vi "Read Measurement Units.vi"(7 "Unit ID (A)":string="A", 8 "error in":errorcluster, 10 "Software Rev":u8, 11 "VISA Session In":refnum<visa-resource-name>="Alicat") -> (0 "error out":errorcluster, 1 "Lock Gas Select":bool, 2 "Measurement Units":T2, 3 "VISA Session Out":refnum<visa-resource-name>)   [LabVIEW 2016]
doc: "Reads the measurement units for the available variables. Measurement units are returned as strings."
uses:
  Omega FMA-1600A Series Gas Flow Meter/Type Definitions/FMA1600A Units String.ctl
  Omega FMA-1600A Series Gas Flow Meter/Type Definitions/FMA1600A Units.ctl
panel:
  in  "Gauge (T) or \nDifferential (F)":bool
  out "Measurement Units Intermediate\n(newer revisions)":T1={"Abs. Pressure Units"=1, "Gauge/Diff. Press. Units"=1, "Barometric Press. Units"=1, "Temperature Units"=1, "Volumetric Units"=1, "Mass Units"=1, "Setpoint Units"=1, "Valve Drive Units"=1, "Total Mass Units"=1, "Total Volume Units"=1, "Time Units"=1} {"Setpoint Units" items=["Default"=0, "Unknown"=1, "SuL/m"=2, "SmL/s"=3, "SmL/m"=4, "SmL/h"=5, "SL/s"=6, "SLPM"=7, "SL/h"=8, "SCCS"=11, "SCCM"=12, "Scm3/h"=13, "Sm3/m"=14, "Sm3/h"=15, "Sm3/d"=16, "Sin3/m"=17, "SCFM"=18, "SCFH"=19, "kSCFM"=20, "NuL/m"=32, "NmL/s"=33, "NmL/m"=34, "NmL/h"=35, "NL/s"=36, "NLPM"=37, "NL/h"=38, "NCCS"=41, "NCCM"=42, "Ncm3/h"=43, "Nm3/m"=44, "Nm3/h"=45, "Nm3/d"=46, "count"=62, "%"=63, "mg/s"=64, "mg/m"=65, "g/s"=66, "g/m"=67, "g/h"=68, "kg/m"=69, "kg/h"=70, "oz/s"=71, "oz/m"=72, "lb/m"=73, "lb/h"=74]; "Barometric Press. Units" items=["Default"=0, "Unknown"=1, "Pa"=2, "hPa"=3, "kPa"=4, "MPa"=5, "mbar"=6, "bar"=7, "g/cm2"=8, "kg/cm"=9, "PSI"=10, "PSF"=11, "mTorr"=12, "torr"=13, "mmHg"=14, "inHg"=15, "mmH2O"=16, "mmH2O"=17, "cmH2O"=18, "cmH2O"=19, "inH2O"=20, "inH2O"=21, "atm"=22, "m asl"=23, "ft asl"=24, "V"=61, "count"=62, "%"=63]; "Gauge/Diff. Press. Units" items=["Default"=0, "Unknown"=1, "Pa"=2, "hPa"=3, "kPa"=4, "MPa"=5, "mbar"=6, "bar"=7, "g/cm2"=8, "kg/cm"=9, "PSI"=10, "PSF"=11, "mTorr"=12, "torr"=13, "mmHg"=14, "inHg"=15, "mmH2O"=16, "mmH2O"=17, "cmH2O"=18, "cmH2O"=19, "inH2O"=20, "inH2O"=21, "atm"=22, "m asl"=23, "ft asl"=24, "V"=61, "count"=62, "%"=63]; "Time Units" items=["Default", "Unknown", "h:m:s", "ms", "s", "m", "hour", "day"]; "Total Volume Units" items=["Default"=0, "Unknown"=1, "uL"=2, "mL"=3, "L"=4, "US GAL"=5, "cm3"=6, "m3"=7, "in3"=8, "ft3"=9, "uP"=61]; "Total Mass Units" items=["Default"=0, "Unknown"=1, "SuL"=2, "SmL"=3, "SL"=4, "Scm3"=6, "Sm3"=7, "Sin3"=8, "Sft3"=9, "kSft3"=10, "NuL"=32, "NmL"=33, "NL"=34, "Ncm3"=35, "Nm3"=36, "mg"=64, "g"=65, "kg"=66, "oz"=67, "lb"=68]; "Valve Drive Units" items=["Default"=0, "Unknown"=1, "count"=2, "%"=63]; "Mass Units" items=["Default"=0, "Unknown"=1, "SuL/m"=2, "SmL/s"=3, "SmL/m"=4, "SmL/h"=5, "SL/s"=6, "SLPM"=7, "SL/h"=8, "SCCS"=11, "SCCM"=12, "Scm3/h"=13, "Sm3/m"=14, "Sm3/h"=15, "Sm3/d"=16, "Sin3/m"=17, "SCFM"=18, "SCFH"=19, "kSCFM"=20, "NuL/m"=32, "NmL/s"=33, "NmL/m"=34, "NmL/h"=35, "NL/s"=36, "NLPM"=37, "NL/h"=38, "NCCS"=41, "NCCM"=42, "Ncm3/h"=43, "Nm3/m"=44, "Nm3/h"=45, "Nm3/d"=46, "count"=62, "%"=63, "mg/s"=64, "mg/m"=65, "g/s"=66, "g/m"=67, "g/h"=68, "kg/m"=69, "kg/h"=70, "oz/s"=71, "oz/m"=72, "lb/m"=73, "lb/h"=74]; "Volumetric Units" items=["Default"=0, "Unknown"=1, "uL/m"=2, "mL/s"=3, "mL/m"=4, "mL/h"=5, "L/s"=6, "LPM"=7, "L/h"=8, "US GPM"=9, "US GPH"=10, "CCS"=11, "CCM"=12, "cm3/h"=13, "m3/m"=14, "m3/h"=15, "m3/d"=16, "in3/m"=17, "CFM"=18, "CFH"=19, "count"=62, "%"=63]; "Temperature Units" items=["Default", "Unknown", "°C", "°F", "K", "°Ra"]; "Abs. Pressure Units" items=["Default"=0, "Unknown"=1, "Pa"=2, "hPa"=3, "kPa"=4, "MPa"=5, "mbar"=6, "bar"=7, "g/cm2"=8, "kg/cm"=9, "PSI"=10, "PSF"=11, "mTorr"=12, "torr"=13, "mmHg"=14, "inHg"=15, "mmH2O"=16, "mmH2O"=17, "cmH2O"=18, "cmH2O"=19, "inH2O"=20, "inH2O"=21, "atm"=22, "m asl"=23, "ft asl"=24, "V"=61, "count"=62, "%"=63]}
  out "Measurement Units Intermediate\n(older revisions)":T3={"Pressure Units"=0, "Mass Units"=0, "Temperature Units"=0, "Volume Units"=0, "Totalizer Units"=15, "Totalizer Avg Units"=15} {"Totalizer Units" items=["CC", "uL", "L", "CI", "CF", "CM", "GAL", "mL", "uP", "Lbs", "N/A", "N/A", "N/A", "SCC", "SuL", "SL", "SCI", "SCF", "NCM", "Grams", "Kg", "Lbs", "mg", "SCM", "SmL", "KSCF"]; "Totalizer Avg Units" items=["CCM", "uLPM", "LPM", "CIM", "CFM", "CM/M", "GAL/M", "mLPM", "uP/M", "Lbs/M", "N/A", "N/A", "N/A", "SCCM", "SuLPM", "SLPM", "SCIM", "SCFM", "NCM/M", "Grams/M", "Kg/M", "Lbs/M", "mg/M", "SCM/M", "SmLPM", "KSCFM"]; "Volume Units" items=["CCM"=0, "CCH"=64, "uLPM"=256, "LPS"=320, "LPM"=512, "CM/D"=576, "CIM"=768, "Percent"=832, "CFH"=1024, "Kg/M"=1088, "CM/H"=1280, "Kg/H"=1344, "CFM"=1536, "mLPS"=1600, "GPM"=1792, "CCS"=1856, "GPH"=2048, "mLPH"=2112, "Grams/S"=2304, "Lbs/H"=2368, "Grams/M"=2560, "Grams/H"=2816, "mg/M"=3072, "LPH"=3328, "oz/S"=3584, "mLPM"=3840]; "Temperature Units" items=["C"=0, "K"=16, "F"=32, "R"=48]; "Mass Units" items=["SCCM"=0, "SLPH"=128, "SuLPM"=4096, "SmLPM"=4224, "SLPM"=8192, "Grams/S"=8320, "SCIM"=12288, "SCM/H"=12416, "SCFH"=16384, "SCCH"=16512, "NCM/H"=20480, "NLPH"=20608, "SCFM"=24576, "NLPS"=24704, "Grams/M"=28672, "SCM/D"=28800, "Grams/H"=32768, "NmLPM"=32896, "Kg/M"=36864, "SCCS"=36992, "Kg/H"=40960, "NmLPH"=41088, "Lbs/M"=45056, "SLPS"=45184, "Lbs/H"=49152, "SmLPS"=49280, "mg/M"=53248, "mg/S"=53376, "NLPM"=57344, "NCCM"=61440]; "Pressure Units" items=["PSI", "PSI", "Torr", "Bar", "mBar", "Pascal", "KPa", "MPa", "inHg", "mmHg", "inH2O", "PSID", "mTorr", "cmH2O", "Kg/CM2", "mmH2O"]}
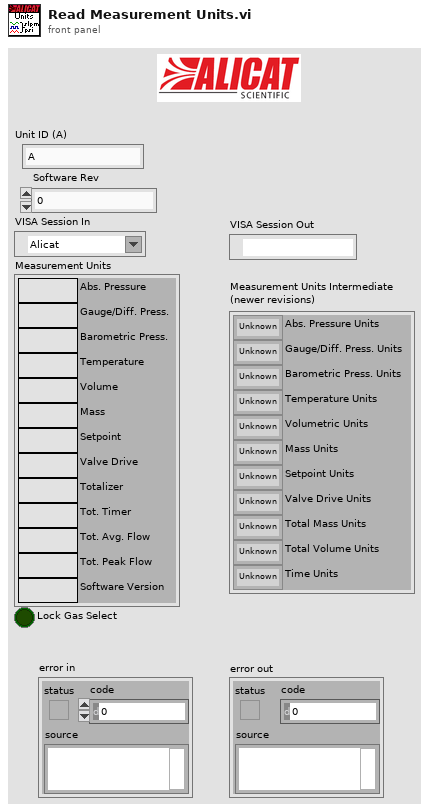
[diagram p1: front panel]
types:
  T1 = typedef "FMA1600A Units.ctl" = cluster{"Abs. Pressure Units":u16, "Gauge/Diff. Press. Units":u16, "Barometric Press. Units":u16, "Temperature Units":u16, "Volumetric Units":u16, "Mass Units":u16, "Setpoint Units":u16, "Valve Drive Units":u16, "Total Mass Units":u16, "Total Volume Units":u16, "Time Units":u16}
  T2 = typedef "FMA1600A Units String.ctl" = cluster{"Abs. Pressure":string, "Gauge/Diff. Press.":string, "Barometric Press.":string, "Temperature":string, "Volume":string, "Mass":string, "Setpoint":string, "Valve Drive":string, "Totalizer":string, "Tot. Timer":string, "Tot. Avg. Flow":string, "Tot. Peak Flow":string, "Software Version":string}
  T3 = cluster{"Pressure Units":i32, "Mass Units":i32, "Temperature Units":i32, "Volume Units":i32, "Totalizer Units":u16, "Totalizer Avg Units":u16}
  T4 = cluster{"Pressure":i32, "Mass":i32, "Temperature":i32, "Volume":i32, "Totalizer Units":u16, "Totalizer Avg Units":u16}
  T5 = typedef "LVStringsAndValuesArrayTypeDef_U16.ctl" = cluster{"String":string, "Value":u16}[]
  T6 = cluster{"Controller Select":u16, "SetPoint Source":enum8{"Serial", "Local", "Analog", "Unknown"}, "AutoTare":enum16{"Disabled", "Enabled"}}
  T7 = typedef "LVStringsAndValuesArrayTypeDef_I32.ctl" = cluster{"String":string, "Value":i32}[]
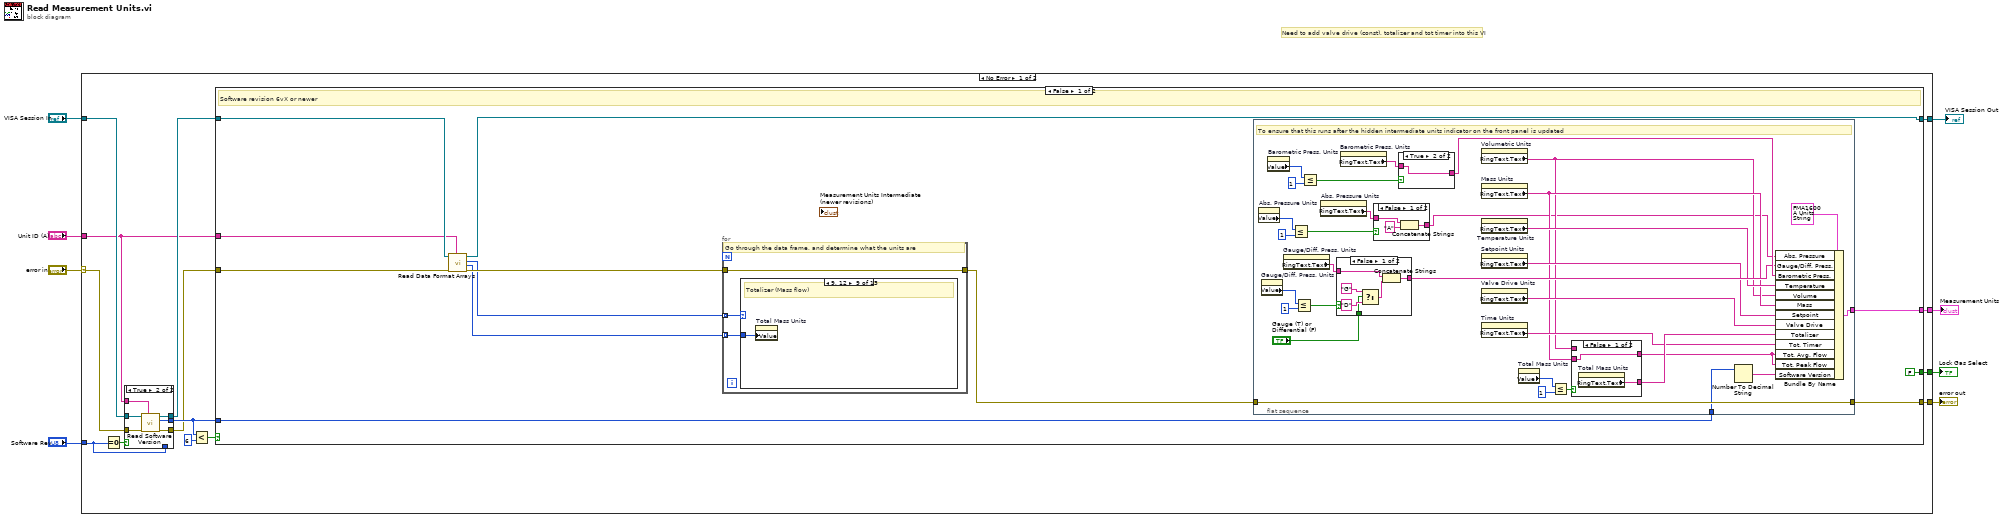
[diagram p0: block diagram]
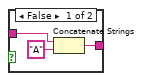
[diagram p4: hidden frame]
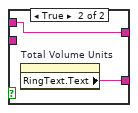
[diagram p6: hidden frame]
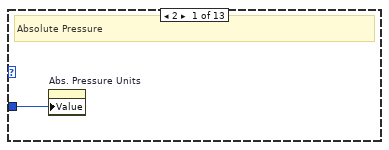
[diagram p7: hidden frame]
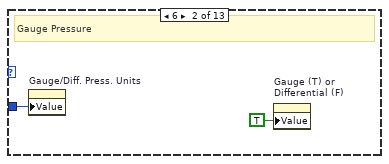
[diagram p8: hidden frame]
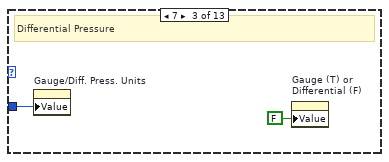
[diagram p9: hidden frame]
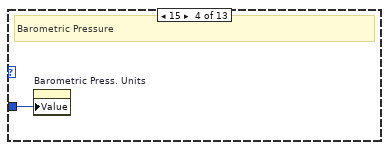
[diagram p10: hidden frame]
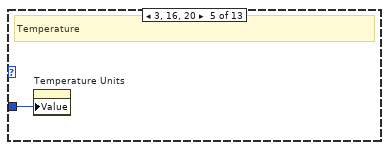
[diagram p11: hidden frame]
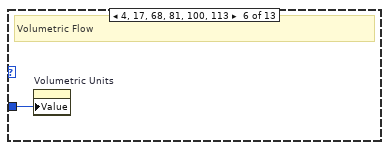
[diagram p12: hidden frame]
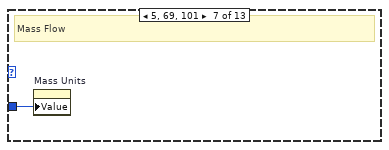
[diagram p13: hidden frame]
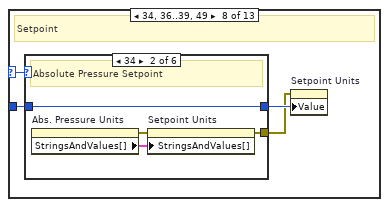
[diagram p14: hidden frame]
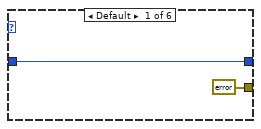
[diagram p15: hidden frame]
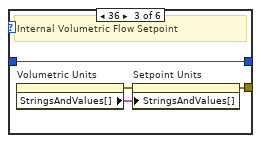
[diagram p16: hidden frame]
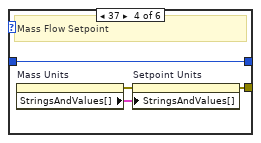
[diagram p17: hidden frame]
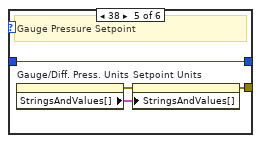
[diagram p18: hidden frame]
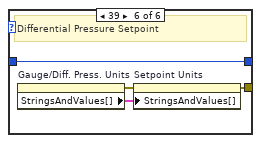
[diagram p19: hidden frame]
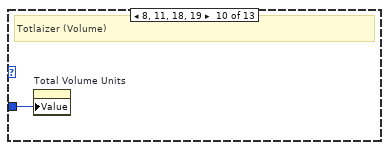
[diagram p20: hidden frame]
diagram:
  # "Need to add valve drive (const), totalizer and tot timer into this VI"
  n1 = case shown="No Error" "error in" {
    selector: "error in" -> [w11 w259]
    tunnel: [w22 TRUE ("Lock Gas Select")] -> w8
    tunnel: [w21 w259] -> w7
    tunnel: "Software Rev" -> [w15 _]
    tunnel: "Unit ID (A)" -> [w9 _]
    tunnel: "VISA Session In" -> [w10 w261]
    tunnel: [w19 w261] -> w3
    tunnel: [w18 T2 {"Abs. Pressure"="PSIA", "Gauge/Diff. Press."="Unknown", "Barometric Press."="Unknown", "Temperature"="°F", "Volume"="LPM", "Mass"="SLPM", "Setpoint"="Unknown", "Valve Drive"="Unknown", "Totalizer"="SL", "Tot. Timer"="Unknown", "Tot. Avg. Flow"="SLPM", "Tot. Peak Flow"="SLPM", "Software Version"=""} ("Measurement Units 2")] -> w2
    frame No Error {
      n2 = Equal To 0?(x=w15) -> (x = 0?=w16:bool)
      n3 = case shown="True" w16 {
        tunnel: w11 -> [w24 w31]
        tunnel: w10 -> [w23 w30]
        tunnel: w9 -> [_ w29]
        tunnel: [w24 w28] -> w12
        tunnel: [w23 w27] -> w13
        tunnel: [w25 w26] -> w14
        tunnel: w15 -> [w25 _]
        frame False {
        }
        frame True {
          n4 = call "Read Software Version.vi"("Unit ID (A)"=w29, "error in"=w31, "VISA Session In"=w30) -> ("error out"=w28:errorcluster, "Software Version"=w26:u8, "VISA Session Out"=w27:refnum<visa-resource-name>)  [unwired: 6 in]
        }
      }
      n5 = Less?(x=w14, y=u8 6) -> (x < y?=w20:bool)
      n6 = case shown="False" w20 {
        tunnel: [FALSE ("Lock Gas Select") w160] -> w22
        tunnel: w12 -> [w39 w152]
        tunnel: [w41 w147] -> w21
        tunnel: w14 -> [w32 w137]
        tunnel: w13 -> [w38 w153]
        tunnel: w9 -> [w37 w142]
        tunnel: [w36 w149] -> w19
        tunnel: [w40 w148] -> w18
        frame False {
          # "Software revision 6vX or newer"
          n7 = call "Read Data Format Arrays.vi"("Unit ID (A)"=w37, "error in (no error)"=w39, "VISA Session In"=w38) -> ("error out"=w35:errorcluster, "Units Array"=w33:u16[], "Data Type Array"=w34:u16[], "VISA Session Out"=w36:refnum<visa-resource-name>)  [unwired: 5 in]
          n8 = for {
            tunnel: w33 -> [w96] mode=indexing
            tunnel: w34 -> [w97] mode=indexing
            tunnel: [w95] -> w42
            tunnel: w35 -> [w95]
            # "Go through the data frame, and determine what the units are"
            n9 = case shown="9, 12" w97 {
              selector: w97 -> [_ _ _ _ _ _ _ w108 _ _ _ _ _]
              tunnel: w96 -> [w98 w100 w102 w103 w104 w105 w106 w107 w133 w134 w135 w136 _]
              frame 2 {
                # "Absolute Pressure"
                n10 = property on="Abs. Pressure Units" class="Ring (strict)"("Value"=w98) -> ()  [unwired: 2 in, 2 out]
              }
              frame 6 {
                # "Gauge Pressure"
                n11 = property on="Gauge/Diff. Press. Units" class="Ring (strict)"("Value"=w100) -> ()  [unwired: 2 in, 2 out]
                n12 = property on="Gauge (T) or \nDifferential (F)" class="Bool (strict)"("Value"=TRUE ("Gauge")) -> ()  [unwired: 2 in, 2 out]
              }
              frame 7 {
                # "Differential Pressure"
                n13 = property on="Gauge/Diff. Press. Units" class="Ring (strict)"("Value"=w102) -> ()  [unwired: 2 in, 2 out]
                n14 = property on="Gauge (T) or \nDifferential (F)" class="Bool (strict)"("Value"=FALSE ("Gauge")) -> ()  [unwired: 2 in, 2 out]
              }
              frame 15 {
                # "Barometric Pressure"
                n15 = property on="Barometric Press. Units" class="Ring (strict)"("Value"=w103) -> ()  [unwired: 2 in, 2 out]
              }
              frame 3, 16, 20 {
                # "Temperature"
                n16 = property on="Temperature Units" class="Ring (strict)"("Value"=w104) -> ()  [unwired: 2 in, 2 out]
              }
              frame 4, 17, 68, 81, 100, 113 {
                # "Volumetric Flow"
                n17 = property on="Volumetric Units" class="Ring (strict)"("Value"=w105) -> ()  [unwired: 2 in, 2 out]
              }
              frame 5, 69, 101 {
                # "Mass Flow"
                n18 = property on="Mass Units" class="Ring (strict)"("Value"=w106) -> ()  [unwired: 2 in, 2 out]
              }
              frame 34, 36..39, 49 {
                # "Setpoint"
                n19 = case shown="34" w108 {
                  tunnel: [w111 w113 w117 w121 w125 w129] -> w110
                  tunnel: [errorcluster {"status"=FALSE, "code"=0, "source"=""} ("error out") w114 w118 w122 w126 w130] -> w109
                  tunnel: w107 -> [w111 w113 w117 w121 w125 w129]
                  frame Default {
                  }
                  frame 34 {
                    # "Absolute Pressure Setpoint"
                    n20 = property on="Abs. Pressure Units" class="Ring (strict)"() -> (error out=w116:errorcluster, "StringsAndValues[]"=w115:T5)  [unwired: 2 in, 1 out]
                    n21 = property on="Setpoint Units" class="Ring (strict)"(error in=w116, "StringsAndValues[]"=w115) -> (error out=w114:errorcluster)  [unwired: 1 in, 1 out]
                  }
                  frame 36 {
                    # "Internal Volumetric Flow Setpoint"
                    n22 = property on="Volumetric Units" class="Ring (strict)"() -> (error out=w120:errorcluster, "StringsAndValues[]"=w119:T5)  [unwired: 2 in, 1 out]
                    n23 = property on="Setpoint Units" class="Ring (strict)"(error in=w120, "StringsAndValues[]"=w119) -> (error out=w118:errorcluster)  [unwired: 1 in, 1 out]
                  }
                  frame 37 {
                    # "Mass Flow Setpoint"
                    n24 = property on="Mass Units" class="Ring (strict)"() -> (error out=w124:errorcluster, "StringsAndValues[]"=w123:T5)  [unwired: 2 in, 1 out]
                    n25 = property on="Setpoint Units" class="Ring (strict)"(error in=w124, "StringsAndValues[]"=w123) -> (error out=w122:errorcluster)  [unwired: 1 in, 1 out]
                  }
                  frame 38 {
                    # "Gauge Pressure Setpoint"
                    n26 = property on="Gauge/Diff. Press. Units" class="Ring (strict)"() -> (error out=w128:errorcluster, "StringsAndValues[]"=w127:T5)  [unwired: 2 in, 1 out]
                    n27 = property on="Setpoint Units" class="Ring (strict)"(error in=w128, "StringsAndValues[]"=w127) -> (error out=w126:errorcluster)  [unwired: 1 in, 1 out]
                  }
                  frame 39 {
                    # "Differential Pressure Setpoint"
                    n28 = property on="Gauge/Diff. Press. Units" class="Ring (strict)"() -> (error out=w132:errorcluster, "StringsAndValues[]"=w131:T5)  [unwired: 2 in, 1 out]
                    n29 = property on="Setpoint Units" class="Ring (strict)"(error in=w132, "StringsAndValues[]"=w131) -> (error out=w130:errorcluster)  [unwired: 1 in, 1 out]
                  }
                }
                n30 = property on="Setpoint Units" class="Ring (strict)"(error in=w109, "Value"=w110) -> ()  [unwired: 1 in, 2 out]
              }
              frame 9, 12 {
                # "Totalizer (Mass flow)"
                n31 = property on="Total Mass Units" class="Ring (strict)"("Value"=w133) -> ()  [unwired: 2 in, 2 out]
              }
              frame 8, 11, 18, 19 {
                # "Totlaizer (Volume)"
                n32 = property on="Total Volume Units" class="Ring (strict)"("Value"=w134) -> ()  [unwired: 2 in, 2 out]
              }
              frame 13 {
                # "Valve Drive"
                n33 = property on="Valve Drive Units" class="Ring (strict)"("Value"=w135) -> ()  [unwired: 2 in, 2 out]
              }
              frame 10, 14 {
                # "Time"
                n34 = property on="Time Units" class="Ring (strict)"("Value"=w136) -> ()  [unwired: 2 in, 2 out]
              }
              frame Default {
              }
            }
          }
          n35 = flat-sequence {
            tunnel: w42 -> [w62]
            tunnel: [w62] -> w41
            tunnel: [w48] -> w40
            tunnel: w32 -> [w45]
            frame #0 {
              # "To ensure that this runs after the hidden intermediate units indicator on the front panel is updated"
              n36 = property on="Abs. Pressure Units" class="Ring (strict)"() -> ("Value"=w68:u16)  [unwired: 2 in, 2 out]
              n37 = property on="Gauge/Diff. Press. Units" class="Ring (strict)"() -> ("Value"=w69:u16)  [unwired: 2 in, 2 out]
              n38 = property on="Barometric Press. Units" class="Ring (strict)"() -> ("Value"=w72:u16)  [unwired: 2 in, 2 out]
              n39 = property on="Gauge/Diff. Press. Units" class="Ring (strict)"() -> ("RingText.Text"=w59:string)  [unwired: 2 in, 2 out]
              n40 = Less Or Equal?(x=w68, y=u16 1) -> (x <= y?=w66:bool)
              n41 = Less Or Equal?(x=w69, y=u16 1) -> (x <= y?=w60:bool)
              n42 = Less Or Equal?(x=w72, y=u16 1) -> (x <= y?=w63:bool)
              n43 = property on="Abs. Pressure Units" class="Ring (strict)"() -> ("RingText.Text"=w65:string)  [unwired: 2 in, 2 out]
              n44 = case shown="False" w60 {
                tunnel: w59 -> [w81 w82]
                tunnel: [w80 w82] -> w57
                tunnel: "Gauge (T) or \nDifferential (F)" -> [w76 _]
                frame False {
                  n45 = Select(t="G" ("string"), s=w76, f="D" ("string")) -> (s? t:f=w77:string)
                  n46 = Concatenate Strings(w81, w77) -> (w80:string)
                }
                frame True {
                }
              }
              n47 = property on="Barometric Press. Units" class="Ring (strict)"() -> ("RingText.Text"=w64:string)  [unwired: 2 in, 2 out]
              n48 = case shown="False" w66 {
                tunnel: w65 -> [w88 w90]
                tunnel: [w87 w90] -> w47
                frame False {
                  n49 = Concatenate Strings(w88, "A" ("string")) -> (w87:string)
                }
                frame True {
                }
              }
              n50 = case shown="True" w63 {
                tunnel: w64 -> [w84 w86]
                tunnel: [w83 w86] -> w58
                frame False {
                  n51 = Concatenate Strings(w84, "A" ("string")) -> (w83:string)
                }
                frame True {
                }
              }
              n52 = property on="Volumetric Units" class="Ring (strict)"() -> ("RingText.Text"=w50:string)  [unwired: 2 in, 2 out]
              n53 = property on="Mass Units" class="Ring (strict)"() -> ("RingText.Text"=w51:string)  [unwired: 2 in, 2 out]
              n54 = property on="Temperature Units" class="Ring (strict)"() -> ("RingText.Text"=w56:string)  [unwired: 2 in, 2 out]
              n55 = property on="Setpoint Units" class="Ring (strict)"() -> ("RingText.Text"=w54:string)  [unwired: 2 in, 2 out]
              n56 = property on="Valve Drive Units" class="Ring (strict)"() -> ("RingText.Text"=w53:string)  [unwired: 2 in, 2 out]
              n57 = property on="Time Units" class="Ring (strict)"() -> ("RingText.Text"=w52:string)  [unwired: 2 in, 2 out]
              n58 = property on="Total Mass Units" class="Ring (strict)"() -> ("Value"=w73:u16)  [unwired: 2 in, 2 out]
              n59 = Less Or Equal?(x=w73, y=u16 1) -> (x <= y?=w74:bool)
              n60 = case shown="False" w74 {
                tunnel: [w92 w94] -> w55
                tunnel: w51 -> [w91 _]
                tunnel: w50 -> [_ w93]
                tunnel: [w91 w93] -> w49
                frame False {
                  n61 = property on="Total Mass Units" class="Ring (strict)"() -> ("RingText.Text"=w92:string)  [unwired: 2 in, 2 out]
                }
                frame True {
                  n62 = property on="Total Volume Units" class="Ring (strict)"() -> ("RingText.Text"=w94:string)  [unwired: 2 in, 2 out]
                }
              }
              n63 = Number To Decimal String(number=w45) -> (decimal integer string=w44:string)  [unwired: 1 in]
              n64 = Bundle By Name(cluster=T2 {"Abs. Pressure"="PSIA", "Gauge/Diff. Press."="Unknown", "Barometric Press."="Unknown", "Temperature"="°F", "Volume"="LPM", "Mass"="SLPM", "Setpoint"="Unknown", "Valve Drive"="Unknown", "Totalizer"="SL", "Tot. Timer"="Unknown", "Tot. Avg. Flow"="SLPM", "Tot. Peak Flow"="SLPM", "Software Version"=""} ("Measurement Units 2"), "Abs. Pressure"=w47, "Gauge/Diff. Press."=w57, "Barometric Press."=w58, "Temperature"=w56, "Volume"=w50, "Mass"=w51, "Setpoint"=w54, "Valve Drive"=w53, "Totalizer"=w55, "Tot. Timer"=w52, "Tot. Avg. Flow"=w49, "Tot. Peak Flow"=w49, "Software Version"=w44) -> (w48:T2)
            }
          }
        }
        frame True {
          # "If true mass units on an \nold board: lock gas select"
          # "Software revision 5vX or older"
          n65 = call "Read Register.vi"("Unit ID (A)"=w142, "error in"=w152, "Register address"=u16 45, "VISA Session In"=w153) -> ("error out"=w146:errorcluster, "Register Value (I32)"=w151:i32, "VISA Session Out"=w144:refnum<visa-resource-name>)  [unwired: 5 in]
          n66 = call "Read Output Definitions and Controller Options.vi"("Unit ID (A)"=w142, "error in"=w146, "VISA Session In"=w144) -> ("error out"=w145:errorcluster, "Read/Write Options"=w141:T6, "VISA Session Out"=w143:refnum<visa-resource-name>)  [unwired: 5 in, 1 out]
          n67 = Unbundle By Name(w141) -> ("Controller Select"=w140:u16)
          n68 = call "Read Totalizer Units and Decimals.vi"("Unit ID (A)"=w142, "error in"=w145, "VISA Session In"=w143) -> ("error out"=w150:errorcluster, "Totalizer Units"=w139:string, "VISA Session Out"=w149:refnum<visa-resource-name>)  [unwired: 4 in, 2 out]
          n69 = property on="Mass Units" class="Ring (strict)"(error in=w150) -> (error out=w159:errorcluster, "StringsAndValues[]"=w197:T7)  [unwired: 1 in, 1 out]
          n70 = for {
            tunnel: w197 -> [w257] mode=indexing
            tunnel: [w256] -> w173 mode=indexing
            n71 = Unbundle By Name(w257) -> ("Value"=w256:i32)
          }
          n72 = property on="Volume Units" class="Ring (strict)"(error in=w159) -> (error out=w158:errorcluster, "StringsAndValues[]"=w188:T7)  [unwired: 1 in, 1 out]
          n73 = Less Or Equal?(x=w173, y=w151) -> (x <= y?=w196:bool[])
          n74 = Boolean To (0,1)(Boolean=w196) -> (0, 1=w195:i16[])
          n75 = To Long Integer(number=w195) -> (32bit integer=w194:i32[])
          n76 = Multiply(x=w173, y=w194) -> (x*y=w193:i32[])
          n77 = for {
            tunnel: w188 -> [w255] mode=indexing
            tunnel: [w254] -> w171 mode=indexing
            n78 = Unbundle By Name(w255) -> ("Value"=w254:i32)
          }
          n79 = Array Max & Min(array=w193) -> (max value=w167:i32, max index (indices)=w172:i32)  [unwired: 2 out]
          n80 = Subtract(x=w151, y=w167) -> (x-y=w187:i32)
          n81 = property on="Temperature Units" class="Ring (strict)"(error in=w158) -> (error out=w157:errorcluster, "StringsAndValues[]"=w186:T7)  [unwired: 1 in, 1 out]
          n82 = Less Or Equal?(x=w171, y=w187) -> (x <= y?=w189:bool[])
          n83 = Boolean To (0,1)(Boolean=w189) -> (0, 1=w190:i16[])
          n84 = To Long Integer(number=w190) -> (32bit integer=w191:i32[])
          n85 = Multiply(x=w171, y=w191) -> (x*y=w192:i32[])
          n86 = for {
            tunnel: w186 -> [w253] mode=indexing
            tunnel: [w252] -> w170 mode=indexing
            n87 = Unbundle By Name(w253) -> ("Value"=w252:i32)
          }
          n88 = Array Max & Min(array=w192) -> (max value=w166:i32)  [unwired: 3 out]
          n89 = Subtract(x=w187, y=w166) -> (x-y=w176:i32)
          n90 = property on="Pressure Units" class="Ring (strict)"(error in=w157) -> (error out=w156:errorcluster, "StringsAndValues[]"=w177:T7)  [unwired: 1 in, 1 out]
          n91 = Less Or Equal?(x=w170, y=w176) -> (x <= y?=w185:bool[])
          n92 = Boolean To (0,1)(Boolean=w185) -> (0, 1=w184:i16[])
          n93 = To Long Integer(number=w184) -> (32bit integer=w183:i32[])
          n94 = Multiply(x=w170, y=w183) -> (x*y=w182:i32[])
          n95 = for {
            tunnel: w177 -> [w251] mode=indexing
            tunnel: [w250] -> w169 mode=indexing
            n96 = Unbundle By Name(w251) -> ("Value"=w250:i32)
          }
          n97 = Array Max & Min(array=w182) -> (max value=w165:i32)  [unwired: 3 out]
          n98 = Subtract(x=w176, y=w165) -> (x-y=w175:i32)
          n99 = Less Or Equal?(x=w169, y=w175) -> (x <= y?=w178:bool[])
          n100 = Boolean To (0,1)(Boolean=w178) -> (0, 1=w179:i16[])
          n101 = To Long Integer(number=w179) -> (32bit integer=w180:i32[])
          n102 = Multiply(x=w169, y=w180) -> (x*y=w181:i32[])
          n103 = Array Max & Min(array=w181) -> (max value=w164:i32)  [unwired: 3 out]
          n104 = Subtract(x=w175, y=w164) -> (x-y=w174:i32)
          n105 = Not Equal To 0?(x=w174) -> (x != 0?=w168:bool)
          n106 = case shown="True" w168 {
            tunnel: w173 -> [_ w249]
            tunnel: w172 -> [_ w247]
            tunnel: w171 -> [_ w242]
            tunnel: w170 -> [_ w236]
            tunnel: w169 -> [_ w230]
            tunnel: w167 -> [w223 _]
            tunnel: w166 -> [w222 _]
            tunnel: w165 -> [w221 _]
            tunnel: w164 -> [w220 _]
            tunnel: [w223 w225] -> w198
            tunnel: [w222 w229] -> w161
            tunnel: [w221 w228] -> w163
            tunnel: [w220 w227] -> w162
            tunnel: w151 -> [_ w224]
            frame False {
            }
            frame True {
              # "If remainder =/= 0, then the value used a combination of bits and needs to be re-checked"
              n107 = Decrement(x=w247) -> (x-1=w248:i32)
              n108 = Index Array(array=w249, index=w248) -> (element=w225:i32)
              n109 = Subtract(x=w224, y=w225) -> (x-y=w226:i32)
              n110 = Less Or Equal?(x=w242, y=w226) -> (x <= y?=w246:bool[])
              n111 = Boolean To (0,1)(Boolean=w246) -> (0, 1=w245:i16[])
              n112 = To Long Integer(number=w245) -> (32bit integer=w244:i32[])
              n113 = Multiply(x=w242, y=w244) -> (x*y=w243:i32[])
              n114 = Array Max & Min(array=w243) -> (max value=w229:i32)  [unwired: 3 out]
              n115 = Subtract(x=w226, y=w229) -> (x-y=w237:i32)
              n116 = Less Or Equal?(x=w236, y=w237) -> (x <= y?=w238:bool[])
              n117 = Boolean To (0,1)(Boolean=w238) -> (0, 1=w239:i16[])
              n118 = To Long Integer(number=w239) -> (32bit integer=w240:i32[])
              n119 = Multiply(x=w236, y=w240) -> (x*y=w241:i32[])
              n120 = Array Max & Min(array=w241) -> (max value=w228:i32)  [unwired: 3 out]
              n121 = Subtract(x=w237, y=w228) -> (x-y=w231:i32)
              n122 = Less Or Equal?(x=w230, y=w231) -> (x <= y?=w235:bool[])
              n123 = Boolean To (0,1)(Boolean=w235) -> (0, 1=w234:i16[])
              n124 = To Long Integer(number=w234) -> (32bit integer=w233:i32[])
              n125 = Multiply(x=w230, y=w233) -> (x*y=w232:i32[])
              n126 = Array Max & Min(array=w232) -> (max value=w227:i32)  [unwired: 3 out]
            }
          }
          n127 = Bundle By Name(cluster=T4 {"Pressure"=0, "Mass"=0, "Temperature"=0, "Volume"=0, "Totalizer Units"=15, "Totalizer Avg Units"=15} ("Measurement Units Intermediate\n(older revisions)"), "Mass"=w198, "Volume"=w161, "Temperature"=w163, "Pressure"=w162) -> (w155:T4)
          n128 = call "Gas Select Lock Check.vi"("error in"=w156, "Software Rev"=w137, "Volumetric Units Code"=w161, "Mass Units Code"=w198) -> ("error out"=w147:errorcluster, "Lock Gas Select"=w160:bool)  [unwired: 6 in]
          n129 = flat-sequence {
            tunnel: w155 -> [w212]
            tunnel: [w211] -> w148
            tunnel: w140 -> [w210]
            tunnel: w139 -> [w202]
            tunnel: w137 -> [w199]
            frame #0 {
              # "Flat sequence to force this code to execute after the units are determined"
              n130 = property on="Pressure Units" class="Ring (strict)"() -> ("RingText.Text"=w209:string)  [unwired: 2 in, 2 out]
              n131 = property on="Temperature Units" class="Ring (strict)"() -> ("RingText.Text"=w213:string)  [unwired: 2 in, 2 out]
              n132 = property on="Volume Units" class="Ring (strict)"() -> ("RingText.Text"=w208:string)  [unwired: 2 in, 2 out]
              n133 = property on="Mass Units" class="Ring (strict)"() -> ("RingText.Text"=w207:string)  [unwired: 2 in, 2 out]
              n134 = Concatenate Strings(w202, "/M" ("string")) -> (w203:string)
              n135 = case shown="0, Default" w210 {
                tunnel: w209 -> [_ w217 _ _]
                tunnel: w208 -> [_ _ w218 _]
                tunnel: w207 -> [_ _ _ w219]
                tunnel: ["Unknown" ("RingText.Text") w217 w218 w219] -> w206
                frame 0, Default {
                }
                frame 34, 38, 39 {
                }
                frame 36 {
                }
                frame 37 {
                }
              }
              n136 = Number To Decimal String(number=w199) -> (decimal integer string=w200:string)  [unwired: 1 in]
              n137 = Bundle By Name(cluster=T2 {"Abs. Pressure"="PSIA", "Gauge/Diff. Press."="Unknown", "Barometric Press."="Unknown", "Temperature"="°F", "Volume"="LPM", "Mass"="SLPM", "Setpoint"="Unknown", "Valve Drive"="Unknown", "Totalizer"="SL", "Tot. Timer"="Unknown", "Tot. Avg. Flow"="SLPM", "Tot. Peak Flow"="SLPM", "Software Version"=""} ("Measurement Units 2"), "Setpoint"=w206, "Abs. Pressure"=w209, "Gauge/Diff. Press."=w209, "Barometric Press."="N/A", "Temperature"=w213, "Volume"=w208, "Mass"=w207, "Valve Drive"="%", "Totalizer"=w202, "Tot. Avg. Flow"=w203, "Tot. Peak Flow"=w202, "Tot. Timer"="h:m:s", "Software Version"=w200) -> (w211:T2)
              "Measurement Units Intermediate\n(older revisions)" <- w212
            }
          }
        }
      }
    }
    frame Error {
    }
  }
  "error out" <- w7
  "VISA Session Out" <- w3
  "Lock Gas Select" <- w8
  "Measurement Units" <- w2
